vi "0036-Sub_calc_HTU21D.vi"(8 "humi":u8[](array[numeric]), 10 "temp":u8[](array[numeric])) -> (1 "humi":dbl, 3 "temp":dbl)   [LabVIEW 2014]
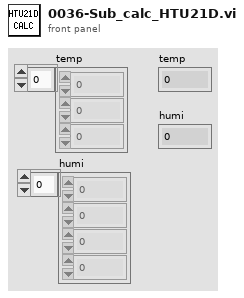
[diagram p1: front panel]
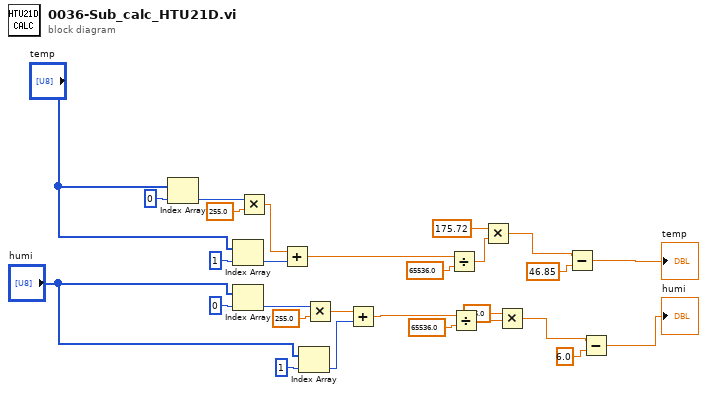
[diagram p0: block diagram]
diagram:
  n1 = Index Array(array="temp", index=0 ("指標")) -> (element=w16:u8)
  n2 = Index Array(array="temp", index=1 ("指標")) -> (element=w19:u8)
  n3 = Index Array(array="humi", index=0 ("指標")) -> (element=w26:u8)
  n4 = Multiply(x=w16, y=255.0) -> (x*y=w18:dbl)
  n5 = Add(x=w18, y=w19) -> (x+y=w10:dbl)
  n6 = Index Array(array="humi", index=1 ("指標")) -> (element=w27:u8)
  n7 = Multiply(x=w26, y=255.0) -> (x*y=w24:dbl)
  n8 = Add(x=w24, y=w27) -> (x+y=w6:dbl)
  n9 = Divide(x=w10, y=65536.0) -> (x/y=w9:dbl)
  n10 = Divide(x=w6, y=65536.0) -> (x/y=w3:dbl)
  n11 = Multiply(x=175.72, y=w9) -> (x*y=w8:dbl)
  n12 = Multiply(x=125.0, y=w3) -> (x*y=w4:dbl)
  n13 = Subtract(x=w8, y=46.85 ("x")) -> (x-y=→"temp":dbl)
  n14 = Subtract(x=w4, y=6.0 ("x")) -> (x-y=→"humi":dbl)
